vi "Log.vi"(8 "error in":errorcluster, 10 "Message":string="Action VI On Recompile was getting called...", 11 "File Name":path=path "ReCompiler.txt") -> (0 "error out":errorcluster)   [LabVIEW 2026]
uses:
  <vilib>/Utility/sysdir.llb/System Directory Type.ctl
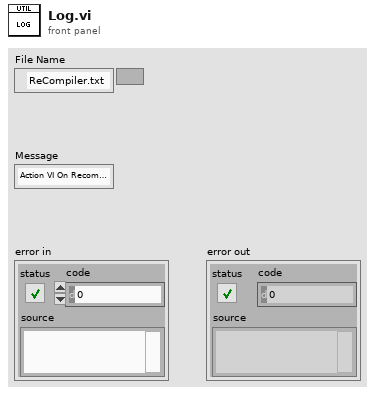
[diagram p1: front panel]
types:
  T1 = enum16{"open", "replace", "create", "open or create", "replace or create", "replace or create with confirmation"}
  T2 = typedef "System Directory Type.ctl" = i32
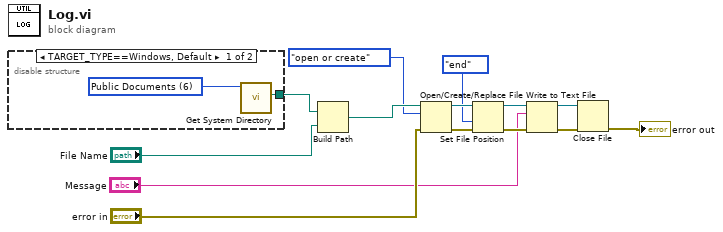
[diagram p0: block diagram]
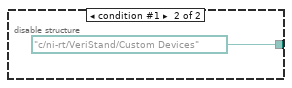
[diagram p2: hidden frame]
diagram:
  n1 = disable-structure shown="TARGET_TYPE==Windows, Default" {
    disable-tunnel: [w15 path "c:/ni-rt/VeriStand/Custom Devices" ("system directory")] -> w9
    frame condition #0 (active) {
      w16 = T2 6 items=["User Home"=0, "User Desktop"=1, "User Documents"=2, "User Application Data"=3, "User Preferences"=4, "User Temporary"=5, "Public Documents"=6, "Public Application Data"=7, "Public Preferences"=8, "Public Cache"=13, "System Core Libraries"=9, "System Installed Libraries"=10, "Application Files"=11, "Boot Volume Root"=12] ("system directory type")
      n2 = call <vilib>:"Get System Directory.vi"("system directory type"=w16) -> ("system directory"=w15:path)  [unwired: 10 in]
    }
    frame condition #1 {
    }
  }
  n3 = Build Path(base path=w9, name or relative path="File Name") -> (appended path=w7:path)
  n4 = Open/Create/Replace File(file path (use dialog)=w7, error in="error in", operation (0:open)=T1."open or create") -> (refnum out=w6:refnum<file>, error out=w14:errorcluster)  [unwired: 3 in, 1 out]
  n5 = Set File Position(refnum=w6, from (0:start)=enum16{"start", "end", "current"}."end", error in=w14) -> (refnum out=w4:refnum<file>, error out=w13:errorcluster)  [unwired: 1 in]
  n6 = Write to Text File(file (use dialog)=w4, text="Message", error in=w13) -> (refnum out=w1:refnum<file>, error out=w11:errorcluster)  [unwired: 1 in, 1 out]
  n7 = Close File(refnum=w1, error in=w11) -> (error out=→"error out":errorcluster)  [unwired: 1 out]
